vi "INIT.vi"(8 "error in (no error)":errorcluster, 11 "SERIAL DEVICE in":refnum<class "SERIAL DEVICE.lvclass">) -> (0 "error out":errorcluster, 3 "SERIAL DEVICE out":refnum<class "SERIAL DEVICE.lvclass">)   [LabVIEW 2019, in "SERIAL DEVICE.lvclass"]
uses:
  SERIAL DEVICE.lvclass
  SERIAL DEVICE.lvclass/SERIAL DEVICE.ctl
  <vilib>/Instr/_visa.llb/VISA Configure Serial Port (Instr).vi
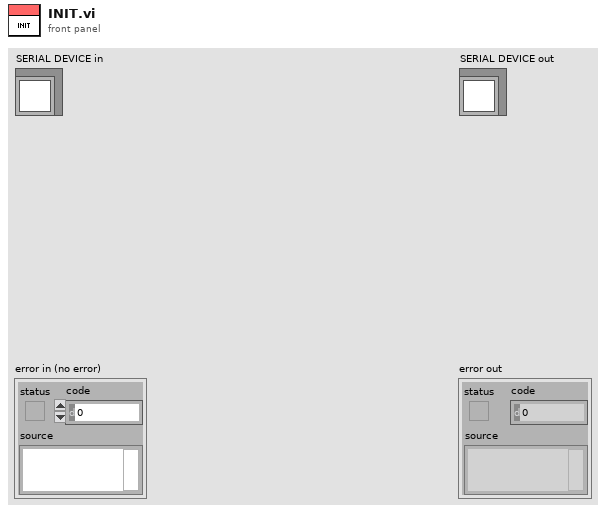
[diagram p1: front panel]
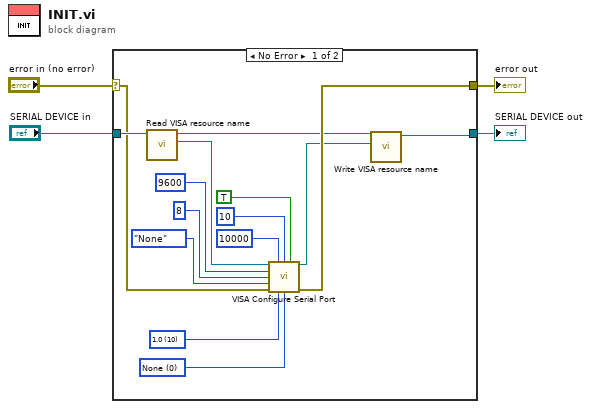
[diagram p0: block diagram]
diagram:
  n1 = case shown="No Error" "error in (no error)" {
    selector: "error in (no error)" -> [w9 w21]
    tunnel: [w8 w21] -> w3
    tunnel: [w6 w20] -> w1
    tunnel: "SERIAL DEVICE in" -> [w19 w20]
    frame No Error {
      w10 = u16 0 items=["None", "XON/XOFF", "RTS/CTS", "XON/XOFF & RTS/CTS", "DTR/DSR", "XON/XOFF & DTR/DSR"] ("flow control (0:none)")
      w11 = u16 10 items=["1.0"=10, "1.5"=15, "2.0"=20] ("stop bits (10: 1 bit)")
      n2 = call "Read VISA resource name.vi"("SERIAL DEVICE in"=w19) -> ("VISA resource name"=w18:refnum<visa-resource-name>, "SERIAL DEVICE out"=w7:refnum<class "SERIAL DEVICE.lvclass">)  [unwired: 8 in, 1 out]
      n3 = call-poly "VISA Configure Serial Port"("VISA resource name"=w18, "timeout (10sec)"=u32 10000, "termination char\n(0xA = '\\n' = LF)"=u8 10 ("termination char\n(0xA = '\\n' = LF)"), "Enable Termination\nChar (T)"=TRUE ("Enable Termination\nChar (T)"), "baud rate (9600)"=u32 9600, "data bits (8)"=u16 8, "parity (0:none)"=enum16{"None", "Odd", "Even", "Mark", "Space"}."None", "error in (no error)"=w9, "stop bits (10: 1 bit)"=w11, "flow control (0:none)"=w10) -> ("VISA resource name out"=w5:refnum<visa-resource-name>, "error out"=w8:errorcluster)  [unwired: 4 in]
      n4 = call "Write VISA resource name.vi"("VISA resource name"=w5, "SERIAL DEVICE in"=w7) -> ("SERIAL DEVICE out"=w6:refnum<class "SERIAL DEVICE.lvclass">)  [unwired: 8 in, 1 out]
    }
    frame Error {
    }
  }
  "error out" <- w3
  "SERIAL DEVICE out" <- w1
